vi "LIN_DBTableToTree.vi"(8 "error in (no error)":errorcluster, 10 "DataBase_array":T1, 11 "reference":refnum<vi>) -> (0 "error out":errorcluster)   [LabVIEW 2014]
uses:
  Typedef/CAN/TCANSignal.ctl
  Typedef/LIN/TLINSignal.ctl
  Typedef/FlexRay/TFlexRaySignal.ctl
  Typedef/TDBSignalProperties.ctl
  Typedef/TDBFrameProperties.ctl
  Typedef/TDBECUProperties.ctl
  Typedef/TDBProperties.ctl
  Typedef/DataBase_array.ctl
  Typedef/DataBase_array_index.ctl
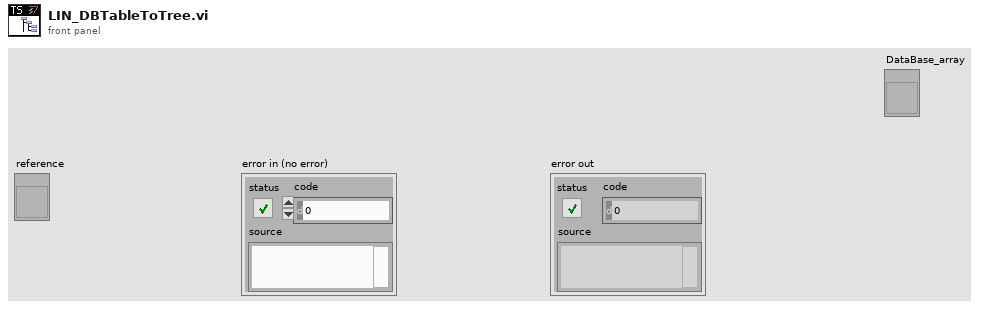
[diagram p1: front panel]
types:
  T1 = typedef "DataBase_array_index.ctl" = refnum<vi>
  T2 = typedef "DataBase_array.ctl" = cluster{"db_properties":T3, "ECU_array":cluster{"TDBECUProperties":T4, "TX_Frame_array":cluster{"Frame_Properties":T5, "signal_array":T6[]}[], "RX_Frame_array":cluster{"Frame_Properties":T5, "signal_array":T6[]}[]}[]}[]
  T3 = typedef "TDBProperties.ctl" = cluster{"FDBIndex":i32, "FSignalCount":i32, "FFrameCount":i32, "FECUCount":i32, "FSupportedChannelMask":u64, "FName":cluster{"数值":u64, "数值 2":u64, "数值 3":u64, "数值 4":u64, "数值 5":u64, "数值 6":u64, "数值 7":u64, "数值 8":u64, "数值 9":u64, "数值 10":u64, "数值 11":u64, "数值 12":u64, "数值 13":u64, "数值 14":u64, "数值 15":u64, "数值 16":u64, "数值 17":u64, "数值 18":u64, "数值 19":u64, "数值 20":u64, "数值 21":u64, "数值 22":u64, "数值 23":u64, "数值 24":u64, "数值 25":u64, "数值 26":u64, "数值 27":u64, "数值 28":u64, "数值 29":u64, "数值 30":u64, "数值 31":u64, "数值 32":u64, "数值 33":u64, "数值 34":u64, "数值 35":u64, "数值 36":u64, "数值 37":u64, "数值 38":u64, "数值 39":u64, "数值 40":u64, "数值 41":u64, "数值 42":u64, "数值 43":u64, "数值 44":u64, "数值 45":u64, "数值 46":u64, "数值 47":u64, "数值 48":u64, "数值 49":u64, "数值 50":u64, "数值 51":u64, "数值 52":u64, "数值 53":u64, "数值 54":u64, "数值 55":u64, "数值 56":u64, "数值 57":u64, "数值 58":u64, "数值 59":u64, "数值 60":u64, "数值 61":u64, "数值 62":u64, "数值 63":u64, "数值 64":u64}, "FComment":cluster{"数值":u64, "数值 2":u64, "数值 3":u64, "数值 4":u64, "数值 5":u64, "数值 6":u64, "数值 7":u64, "数值 8":u64, "数值 9":u64, "数值 10":u64, "数值 11":u64, "数值 12":u64, "数值 13":u64, "数值 14":u64, "数值 15":u64, "数值 16":u64, "数值 17":u64, "数值 18":u64, "数值 19":u64, "数值 20":u64, "数值 21":u64, "数值 22":u64, "数值 23":u64, "数值 24":u64, "数值 25":u64, "数值 26":u64, "数值 27":u64, "数值 28":u64, "数值 29":u64, "数值 30":u64, "数值 31":u64, "数值 32":u64, "数值 33":u64, "数值 34":u64, "数值 35":u64, "数值 36":u64, "数值 37":u64, "数值 38":u64, "数值 39":u64, "数值 40":u64, "数值 41":u64, "数值 42":u64, "数值 43":u64, "数值 44":u64, "数值 45":u64, "数值 46":u64, "数值 47":u64, "数值 48":u64, "数值 49":u64, "数值 50":u64, "数值 51":u64, "数值 52":u64, "数值 53":u64, "数值 54":u64, "数值 55":u64, "数值 56":u64, "数值 57":u64, "数值 58":u64, "数值 59":u64, "数值 60":u64, "数值 61":u64, "数值 62":u64, "数值 63":u64, "数值 64":u64}, "FFlags":u32, "FDBId":u32}
  T4 = typedef "TDBECUProperties.ctl" = cluster{"FDBIndex":i32, "FECUIndex":i32, "FTxFrameCount":i32, "FRxFrameCount":i32, "FName":cluster{"数值":u64, "数值 2":u64, "数值 3":u64, "数值 4":u64, "数值 5":u64, "数值 6":u64, "数值 7":u64, "数值 8":u64, "数值 9":u64, "数值 10":u64, "数值 11":u64, "数值 12":u64, "数值 13":u64, "数值 14":u64, "数值 15":u64, "数值 16":u64, "数值 17":u64, "数值 18":u64, "数值 19":u64, "数值 20":u64, "数值 21":u64, "数值 22":u64, "数值 23":u64, "数值 24":u64, "数值 25":u64, "数值 26":u64, "数值 27":u64, "数值 28":u64, "数值 29":u64, "数值 30":u64, "数值 31":u64, "数值 32":u64, "数值 33":u64, "数值 34":u64, "数值 35":u64, "数值 36":u64, "数值 37":u64, "数值 38":u64, "数值 39":u64, "数值 40":u64, "数值 41":u64, "数值 42":u64, "数值 43":u64, "数值 44":u64, "数值 45":u64, "数值 46":u64, "数值 47":u64, "数值 48":u64, "数值 49":u64, "数值 50":u64, "数值 51":u64, "数值 52":u64, "数值 53":u64, "数值 54":u64, "数值 55":u64, "数值 56":u64, "数值 57":u64, "数值 58":u64, "数值 59":u64, "数值 60":u64, "数值 61":u64, "数值 62":u64, "数值 63":u64, "数值 64":u64}, "FComment":cluster{"数值":u64, "数值 2":u64, "数值 3":u64, "数值 4":u64, "数值 5":u64, "数值 6":u64, "数值 7":u64, "数值 8":u64, "数值 9":u64, "数值 10":u64, "数值 11":u64, "数值 12":u64, "数值 13":u64, "数值 14":u64, "数值 15":u64, "数值 16":u64, "数值 17":u64, "数值 18":u64, "数值 19":u64, "数值 20":u64, "数值 21":u64, "数值 22":u64, "数值 23":u64, "数值 24":u64, "数值 25":u64, "数值 26":u64, "数值 27":u64, "数值 28":u64, "数值 29":u64, "数值 30":u64, "数值 31":u64, "数值 32":u64, "数值 33":u64, "数值 34":u64, "数值 35":u64, "数值 36":u64, "数值 37":u64, "数值 38":u64, "数值 39":u64, "数值 40":u64, "数值 41":u64, "数值 42":u64, "数值 43":u64, "数值 44":u64, "数值 45":u64, "数值 46":u64, "数值 47":u64, "数值 48":u64, "数值 49":u64, "数值 50":u64, "数值 51":u64, "数值 52":u64, "数值 53":u64, "数值 54":u64, "数值 55":u64, "数值 56":u64, "数值 57":u64, "数值 58":u64, "数值 59":u64, "数值 60":u64, "数值 61":u64, "数值 62":u64, "数值 63":u64, "数值 64":u64}}
  T5 = typedef "TDBFrameProperties.ctl" = cluster{"FDBIndex":i32, "FECUIndex":i32, "FFrameIndex":i32, "FIsTx":u8, "FReserved1":u8, "FCycleTimeMs":u16, "TSignalType":i32, "FCANIsDataFrame":u8, "FCANIsStdFrame":u8, "FCANIsEdl":u8, "FCANIsBrs":u8, "FCANIdentifier":i32, "FCANDLC":i32, "FCANDataBytes":i32, "FLINIdentifier":i32, "FLINDLC":i32, "FFRChannelMask":u8, "FFRBaseCycle":u8, "FFRCycleRepetition":u8, "FFRIsStartupFrame":u8, "FFRSlotId":u16, "FFRDLC":u16, "FFRCycleMask":u64, "FSignalCount":i32, "FName":cluster{"数值":u64, "数值 2":u64, "数值 3":u64, "数值 4":u64, "数值 5":u64, "数值 6":u64, "数值 7":u64, "数值 8":u64, "数值 9":u64, "数值 10":u64, "数值 11":u64, "数值 12":u64, "数值 13":u64, "数值 14":u64, "数值 15":u64, "数值 16":u64, "数值 17":u64, "数值 18":u64, "数值 19":u64, "数值 20":u64, "数值 21":u64, "数值 22":u64, "数值 23":u64, "数值 24":u64, "数值 25":u64, "数值 26":u64, "数值 27":u64, "数值 28":u64, "数值 29":u64, "数值 30":u64, "数值 31":u64, "数值 32":u64, "数值 33":u64, "数值 34":u64, "数值 35":u64, "数值 36":u64, "数值 37":u64, "数值 38":u64, "数值 39":u64, "数值 40":u64, "数值 41":u64, "数值 42":u64, "数值 43":u64, "数值 44":u64, "数值 45":u64, "数值 46":u64, "数值 47":u64, "数值 48":u64, "数值 49":u64, "数值 50":u64, "数值 51":u64, "数值 52":u64, "数值 53":u64, "数值 54":u64, "数值 55":u64, "数值 56":u64, "数值 57":u64, "数值 58":u64, "数值 59":u64, "数值 60":u64, "数值 61":u64, "数值 62":u64, "数值 63":u64, "数值 64":u64}, "FComment":cluster{"数值":u64, "数值 2":u64, "数值 3":u64, "数值 4":u64, "数值 5":u64, "数值 6":u64, "数值 7":u64, "数值 8":u64, "数值 9":u64, "数值 10":u64, "数值 11":u64, "数值 12":u64, "数值 13":u64, "数值 14":u64, "数值 15":u64, "数值 16":u64, "数值 17":u64, "数值 18":u64, "数值 19":u64, "数值 20":u64, "数值 21":u64, "数值 22":u64, "数值 23":u64, "数值 24":u64, "数值 25":u64, "数值 26":u64, "数值 27":u64, "数值 28":u64, "数值 29":u64, "数值 30":u64, "数值 31":u64, "数值 32":u64, "数值 33":u64, "数值 34":u64, "数值 35":u64, "数值 36":u64, "数值 37":u64, "数值 38":u64, "数值 39":u64, "数值 40":u64, "数值 41":u64, "数值 42":u64, "数值 43":u64, "数值 44":u64, "数值 45":u64, "数值 46":u64, "数值 47":u64, "数值 48":u64, "数值 49":u64, "数值 50":u64, "数值 51":u64, "数值 52":u64, "数值 53":u64, "数值 54":u64, "数值 55":u64, "数值 56":u64, "数值 57":u64, "数值 58":u64, "数值 59":u64, "数值 60":u64, "数值 61":u64, "数值 62":u64, "数值 63":u64, "数值 64":u64}}
  T6 = typedef "TDBSignalProperties.ctl" = cluster{"FDBIndex":i32, "FECUIndex":i32, "FFrameIndex":i32, "FSignalIndex":i32, "FIsTx":u8, "FReserved1":u8, "FReserved2":u8, "FReserved3":u8, "TSignalType":i32, "TCANSignal":T7, "TLINSignal":T8, "TFlexRaySignal":T9, "FParentFrameId":i32, "FInitValue":dbl, "FName":cluster{"数值":u64, "数值 2":u64, "数值 3":u64, "数值 4":u64, "数值 5":u64, "数值 6":u64, "数值 7":u64, "数值 8":u64, "数值 9":u64, "数值 10":u64, "数值 11":u64, "数值 12":u64, "数值 13":u64, "数值 14":u64, "数值 15":u64, "数值 16":u64, "数值 17":u64, "数值 18":u64, "数值 19":u64, "数值 20":u64, "数值 21":u64, "数值 22":u64, "数值 23":u64, "数值 24":u64, "数值 25":u64, "数值 26":u64, "数值 27":u64, "数值 28":u64, "数值 29":u64, "数值 30":u64, "数值 31":u64, "数值 32":u64, "数值 33":u64, "数值 34":u64, "数值 35":u64, "数值 36":u64, "数值 37":u64, "数值 38":u64, "数值 39":u64, "数值 40":u64, "数值 41":u64, "数值 42":u64, "数值 43":u64, "数值 44":u64, "数值 45":u64, "数值 46":u64, "数值 47":u64, "数值 48":u64, "数值 49":u64, "数值 50":u64, "数值 51":u64, "数值 52":u64, "数值 53":u64, "数值 54":u64, "数值 55":u64, "数值 56":u64, "数值 57":u64, "数值 58":u64, "数值 59":u64, "数值 60":u64, "数值 61":u64, "数值 62":u64, "数值 63":u64, "数值 64":u64}, "FComment":cluster{"数值":u64, "数值 2":u64, "数值 3":u64, "数值 4":u64, "数值 5":u64, "数值 6":u64, "数值 7":u64, "数值 8":u64, "数值 9":u64, "数值 10":u64, "数值 11":u64, "数值 12":u64, "数值 13":u64, "数值 14":u64, "数值 15":u64, "数值 16":u64, "数值 17":u64, "数值 18":u64, "数值 19":u64, "数值 20":u64, "数值 21":u64, "数值 22":u64, "数值 23":u64, "数值 24":u64, "数值 25":u64, "数值 26":u64, "数值 27":u64, "数值 28":u64, "数值 29":u64, "数值 30":u64, "数值 31":u64, "数值 32":u64, "数值 33":u64, "数值 34":u64, "数值 35":u64, "数值 36":u64, "数值 37":u64, "数值 38":u64, "数值 39":u64, "数值 40":u64, "数值 41":u64, "数值 42":u64, "数值 43":u64, "数值 44":u64, "数值 45":u64, "数值 46":u64, "数值 47":u64, "数值 48":u64, "数值 49":u64, "数值 50":u64, "数值 51":u64, "数值 52":u64, "数值 53":u64, "数值 54":u64, "数值 55":u64, "数值 56":u64, "数值 57":u64, "数值 58":u64, "数值 59":u64, "数值 60":u64, "数值 61":u64, "数值 62":u64, "数值 63":u64, "数值 64":u64}}
  T7 = typedef "TCANSignal.ctl" = cluster{"FCANSgnType":u8, "FIsIntel":u8, "FStartBit":i32, "FLength":i32, "FFactor":dbl, "FOffset":dbl}
  T8 = typedef "TLINSignal.ctl" = cluster{"FLINSgnType":u8, "FIsIntel":u8, "FStartBit":i32, "FLength":i32, "FFactor":dbl, "FOffset":dbl}
  T9 = typedef "TFlexRaySignal.ctl" = cluster{"FFRSgnType":u8, "FCompuMethod":u8, "FReserved":u8, "FIsIntel":u8, "FStartBit":i32, "FUpdateBit":i32, "FLength":i32, "FFactor":dbl, "FOffset":dbl, "FActualStartBit":i32, "FActualUpdateBit":i32}
  T10 = cluster{"数值":u64, "数值 2":u64, "数值 3":u64, "数值 4":u64, "数值 5":u64, "数值 6":u64, "数值 7":u64, "数值 8":u64, "数值 9":u64, "数值 10":u64, "数值 11":u64, "数值 12":u64, "数值 13":u64, "数值 14":u64, "数值 15":u64, "数值 16":u64, "数值 17":u64, "数值 18":u64, "数值 19":u64, "数值 20":u64, "数值 21":u64, "数值 22":u64, "数值 23":u64, "数值 24":u64, "数值 25":u64, "数值 26":u64, "数值 27":u64, "数值 28":u64, "数值 29":u64, "数值 30":u64, "数值 31":u64, "数值 32":u64, "数值 33":u64, "数值 34":u64, "数值 35":u64, "数值 36":u64, "数值 37":u64, "数值 38":u64, "数值 39":u64, "数值 40":u64, "数值 41":u64, "数值 42":u64, "数值 43":u64, "数值 44":u64, "数值 45":u64, "数值 46":u64, "数值 47":u64, "数值 48":u64, "数值 49":u64, "数值 50":u64, "数值 51":u64, "数值 52":u64, "数值 53":u64, "数值 54":u64, "数值 55":u64, "数值 56":u64, "数值 57":u64, "数值 58":u64, "数值 59":u64, "数值 60":u64, "数值 61":u64, "数值 62":u64, "数值 63":u64, "数值 64":u64}
  T11 = cluster{"TDBECUProperties":T4, "TX_Frame_array":cluster{"Frame_Properties":T5, "signal_array":T6[]}[], "RX_Frame_array":cluster{"Frame_Properties":T5, "signal_array":T6[]}[]}[]
  T12 = cluster{"Frame_Properties":T5, "signal_array":T6[]}[]
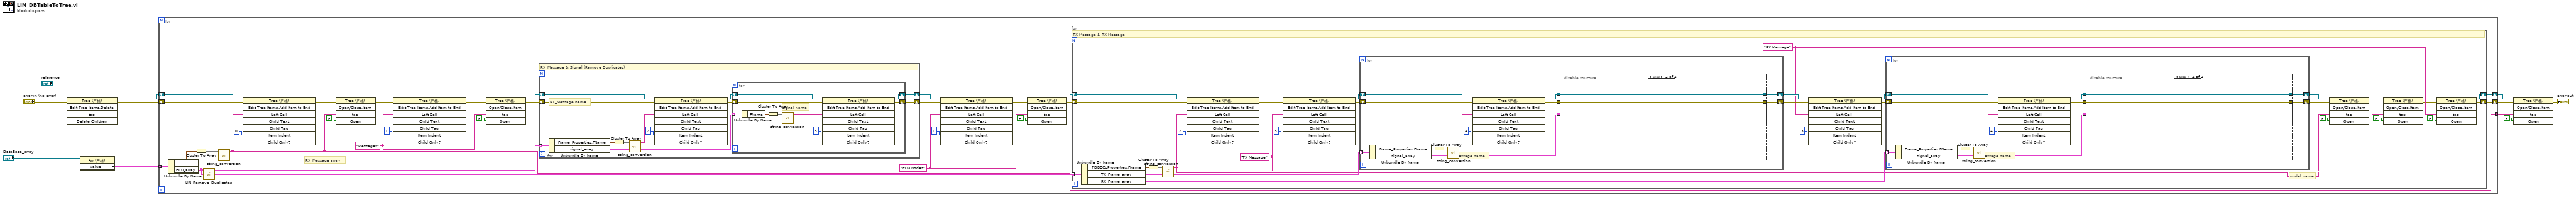
[diagram p0: block diagram]
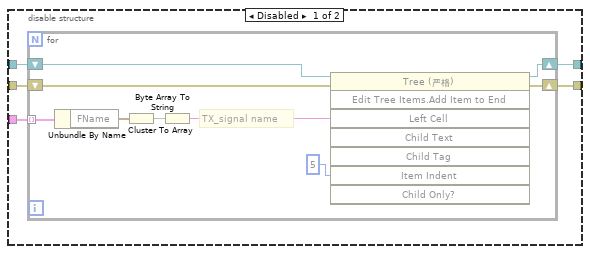
[diagram p2: hidden frame]
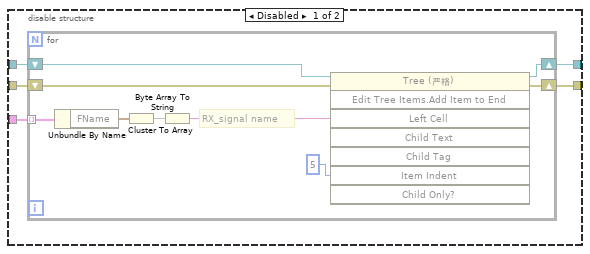
[diagram p3: hidden frame]
diagram:
  n1 = invoke class="Tree (严格)" method="Edit Tree Items.Delete"(reference="reference", error in="error in (no error)") -> (reference out=w11:refnum<vi>, error out=w6:errorcluster)  [unwired: 3 in, 3 out]
  n2 = property class="Arr (严格)"(reference="DataBase_array") -> ("Value"=w2:T2)  [unwired: 1 in, 2 out]
  n3 = for {
    tunnel: [w14] -> w8
    shift-right: [w37] -> w5
    shift-left: w11 -> [w43]
    shift-right: [w36] -> w4
    shift-left: w6 -> [w40]
    tunnel: w2 -> [w29] mode=indexing
    w16 = "Messages" ("Left Cell String")
    w33 = "ECU Nodes" ("Left Cell String")
    # "RX_Message array"
    n4 = Unbundle By Name(w29) -> ("db_properties.FName"=w28:T10, "ECU_array"=w15:T11)
    n5 = Cluster To Array(cluster=w28) -> (array=w12:u64[])
    n6 = call "LIN_Remove_Duplicates.vi"("ECU_array"=w15) -> ("RX_array out"=w13:T12)  [unwired: 10 in]
    n7 = call "string_conversion.vi"("FName"=w12) -> ("string"=w14:string)  [unwired: 10 in]
    n8 = invoke class="Tree (严格)" method="Edit Tree Items.Add Item to End"(reference=w43, error in=w40, "Left Cell"=w14, "Item Indent"=0 ("新项缩进")) -> (reference out=w42:refnum<vi>, error out=w39:errorcluster)  [unwired: 4 in, 6 out]
    n9 = invoke class="Tree (严格)" method="Open/Close.Item"(reference=w42, error in=w39, "tag"=w14, "Open"=FALSE ("Open?")) -> (reference out=w25:refnum<vi>, error out=w24:errorcluster)  [unwired: 1 in, 3 out]
    n10 = invoke class="Tree (严格)" method="Edit Tree Items.Add Item to End"(reference=w25, error in=w24, "Left Cell"=w16, "Item Indent"=1 ("New Item Indentation")) -> (reference out=w20:refnum<vi>, error out=w18:errorcluster)  [unwired: 4 in, 6 out]
    n11 = invoke class="Tree (严格)" method="Open/Close.Item"(reference=w20, error in=w18, "tag"=w16, "Open"=FALSE ("Open?")) -> (reference out=w19:refnum<vi>, error out=w17:errorcluster)  [unwired: 1 in, 3 out]
    n12 = for {
      shift-right: [w55] -> w23
      shift-left: w19 -> [w53]
      shift-right: [w54] -> w22
      shift-left: w17 -> [w52]
      tunnel: w13 -> [w51] mode=indexing
      # "RX_Message name"
      # "RX_Message & Signal (Remove Duplicates)"
      n13 = Unbundle By Name(w51) -> ("Frame_Properties.FName"=w49:T10, "signal_array"=w46:T6[])
      n14 = Cluster To Array(cluster=w49) -> (array=w45:u64[])
      n15 = call "string_conversion.vi"("FName"=w45) -> ("string"=w44:string)  [unwired: 10 in]
      n16 = invoke class="Tree (严格)" method="Edit Tree Items.Add Item to End"(reference=w53, error in=w52, "Left Cell"=w44, "Item Indent"=2 ("New Item Indentation")) -> (reference out=w47:refnum<vi>, error out=w48:errorcluster)  [unwired: 4 in, 6 out]
      n17 = for {
        tunnel: w46 -> [w59] mode=indexing
        shift-right: [w63] -> w55
        shift-left: w47 -> [w64]
        shift-right: [w61] -> w54
        shift-left: w48 -> [w62]
        # "signal name"
        n18 = Unbundle By Name(w59) -> ("FName"=w58:T10)
        n19 = Cluster To Array(cluster=w58) -> (array=w57:u64[])
        n20 = call "string_conversion.vi"("FName"=w57) -> ("string"=w56:string)  [unwired: 10 in]
        n21 = invoke class="Tree (严格)" method="Edit Tree Items.Add Item to End"(reference=w64, error in=w62, "Left Cell"=w56, "Item Indent"=3 ("新项缩进")) -> (reference out=w63:refnum<vi>, error out=w61:errorcluster)  [unwired: 4 in, 6 out]
      }
    }
    n22 = invoke class="Tree (严格)" method="Edit Tree Items.Add Item to End"(reference=w23, error in=w22, "Left Cell"=w33, "Item Indent"=1 ("New Item Indentation")) -> (reference out=w35:refnum<vi>, error out=w31:errorcluster)  [unwired: 4 in, 6 out]
    n23 = invoke class="Tree (严格)" method="Open/Close.Item"(reference=w35, error in=w31, "tag"=w33, "Open"=FALSE ("Open?")) -> (reference out=w34:refnum<vi>, error out=w30:errorcluster)  [unwired: 1 in, 3 out]
    n24 = for {
      shift-right: [w80] -> w37
      shift-left: w34 -> [w95]
      shift-right: [w79] -> w36
      shift-left: w30 -> [w87]
      tunnel: w15 -> [w78] mode=indexing
      w73 = "RX Message" ("Left Cell String")
      w74 = "TX Message" ("Left Cell String")
      # "nodel name"
      # "TX Message & RX Message"
      n25 = Unbundle By Name(w78) -> ("TDBECUProperties.FName"=w77:T10, "TX_Frame_array"=w76:T12, "RX_Frame_array"=w75:T12)
      n26 = Cluster To Array(cluster=w77) -> (array=w66:u64[])
      n27 = call "string_conversion.vi"("FName"=w66) -> ("string"=w65:string)  [unwired: 10 in]
      n28 = invoke class="Tree (严格)" method="Edit Tree Items.Add Item to End"(reference=w95, error in=w87, "Left Cell"=w65, "Item Indent"=2 ("New Item Indentation")) -> (reference out=w93:refnum<vi>, error out=w86:errorcluster)  [unwired: 4 in, 6 out]
      n29 = invoke class="Tree (严格)" method="Edit Tree Items.Add Item to End"(reference=w93, error in=w86, "Left Cell"=w74, "Item Indent"=3 ("New Item Indentation")) -> (reference out=w91:refnum<vi>, error out=w85:errorcluster)  [unwired: 4 in, 6 out]
      n30 = for {
        tunnel: w76 -> [w106] mode=indexing
        shift-right: [w100] -> w88
        shift-left: w91 -> [w107]
        shift-right: [w98] -> w84
        shift-left: w85 -> [w104]
        # "TX_Message name"
        n31 = Unbundle By Name(w106) -> ("Frame_Properties.FName"=w103:T10, "signal_array"=w102:T6[])
        n32 = Cluster To Array(cluster=w103) -> (array=w97:u64[])
        n33 = call "string_conversion.vi"("FName"=w97) -> ("string"=w96:string)  [unwired: 10 in]
        n34 = invoke class="Tree (严格)" method="Edit Tree Items.Add Item to End"(reference=w107, error in=w104, "Left Cell"=w96, "Item Indent"=4 ("New Item Indentation")) -> (reference out=w101:refnum<vi>, error out=w99:errorcluster)  [unwired: 4 in, 6 out]
        n35 = disable-structure shown="启用" {
          disable-tunnel: w102 -> [w112 _]
          disable-tunnel: w101 -> [w111 w123]
          disable-tunnel: [w110 w123] -> w100
          disable-tunnel: w99 -> [w109 w122]
          disable-tunnel: [w108 w122] -> w98
          frame Disabled {
            n36 = for {
              tunnel: w112 -> [w116] mode=indexing
              shift-right: [w120] -> w110
              shift-left: w111 -> [w121]
              shift-right: [w118] -> w108
              shift-left: w109 -> [w119]
              # "TX_signal name"
              n37 = Unbundle By Name(w116) -> ("FName"=w114:T10)
              n38 = Cluster To Array(cluster=w114) -> (array=w115:u64[])
              n39 = Byte Array To String(unsigned byte array=w115) -> (string=w113:string)
              n40 = invoke class="Tree (严格)" method="Edit Tree Items.Add Item to End"(reference=w121, error in=w119, "Left Cell"=w113, "Item Indent"=5 ("新项缩进")) -> (reference out=w120:refnum<vi>, error out=w118:errorcluster)  [unwired: 4 in, 6 out]
            }
          }
          frame Enabled {
          }
        }
      }
      n41 = invoke class="Tree (严格)" method="Edit Tree Items.Add Item to End"(reference=w88, error in=w84, "Left Cell"=w73, "Item Indent"=3 ("New Item Indentation")) -> (reference out=w90:refnum<vi>, error out=w83:errorcluster)  [unwired: 4 in, 6 out]
      n42 = for {
        shift-right: [w127] -> w82
        shift-left: w90 -> [w135]
        shift-right: [w129] -> w81
        shift-left: w83 -> [w133]
        tunnel: w75 -> [w131] mode=indexing
        # "RX_Message name"
        n43 = Unbundle By Name(w131) -> ("Frame_Properties.FName"=w132:T10, "signal_array"=w126:T6[])
        n44 = Cluster To Array(cluster=w132) -> (array=w125:u64[])
        n45 = call "string_conversion.vi"("FName"=w125) -> ("string"=w124:string)  [unwired: 10 in]
        n46 = invoke class="Tree (严格)" method="Edit Tree Items.Add Item to End"(reference=w135, error in=w133, "Left Cell"=w124, "Item Indent"=4 ("New Item Indentation")) -> (reference out=w128:refnum<vi>, error out=w130:errorcluster)  [unwired: 4 in, 6 out]
        n47 = disable-structure shown="启用" {
          disable-tunnel: w130 -> [w140 w150]
          disable-tunnel: [w139 w150] -> w129
          disable-tunnel: w128 -> [w138 w151]
          disable-tunnel: [w137 w151] -> w127
          disable-tunnel: w126 -> [w136 _]
          frame Disabled {
            n48 = for {
              tunnel: w136 -> [w144] mode=indexing
              shift-right: [w148] -> w137
              shift-left: w138 -> [w149]
              shift-right: [w146] -> w139
              shift-left: w140 -> [w147]
              # "RX_signal name"
              n49 = Unbundle By Name(w144) -> ("FName"=w142:T10)
              n50 = Cluster To Array(cluster=w142) -> (array=w143:u64[])
              n51 = Byte Array To String(unsigned byte array=w143) -> (string=w141:string)
              n52 = invoke class="Tree (严格)" method="Edit Tree Items.Add Item to End"(reference=w149, error in=w147, "Left Cell"=w141, "Item Indent"=5 ("新项缩进")) -> (reference out=w148:refnum<vi>, error out=w146:errorcluster)  [unwired: 4 in, 6 out]
            }
          }
          frame Enabled {
          }
        }
      }
      n53 = invoke class="Tree (严格)" method="Open/Close.Item"(reference=w82, error in=w81, "tag"=w65, "Open"=FALSE ("Open?")) -> (reference out=w71:refnum<vi>)  [unwired: 1 in, 4 out]
      n54 = invoke class="Tree (严格)" method="Open/Close.Item"(reference=w71, "tag"=w74, "Open"=FALSE ("Open?")) -> (reference out=w70:refnum<vi>, error out=w69:errorcluster)  [unwired: 2 in, 3 out]
      n55 = invoke class="Tree (严格)" method="Open/Close.Item"(reference=w70, error in=w69, "tag"=w73, "Open"=FALSE ("Open?")) -> (reference out=w80:refnum<vi>, error out=w79:errorcluster)  [unwired: 1 in, 3 out]
    }
  }
  n56 = invoke class="Tree (严格)" method="Open/Close.Item"(reference=w5, error in=w4, "tag"=w8, "Open"=FALSE ("Open?")) -> (error out=→"error out":errorcluster)  [unwired: 1 in, 4 out]
